vi "Get Control Reference.vi"(8 "error in":errorcluster, 9 "Control Label":string, 11 "Front Panel Reference In":refnum<vi>) -> (0 "error out":errorcluster, 1 "Selected Control Reference":refnum<vi>, 2 "Control References Array":refnum<vi>[](array[refnum]), 3 "Front Panel Reference Out":refnum<vi>)   [LabVIEW 2017, in "DTacq Plot Display Library.lvlib"]
uses:
  DTacq Plot Display Library.lvlib
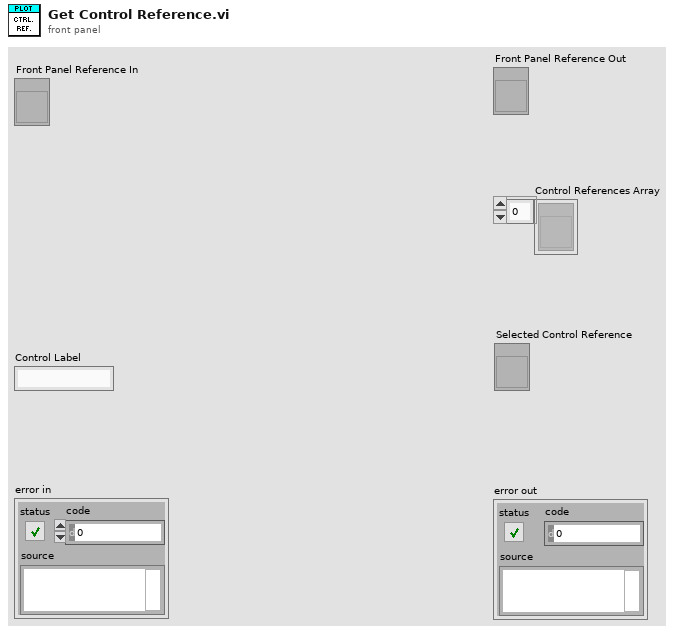
[diagram p1: front panel]
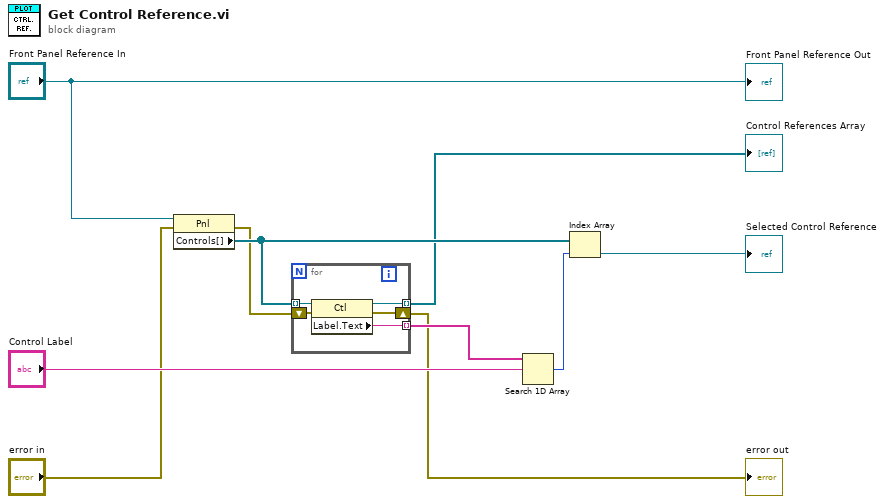
[diagram p0: block diagram]
diagram:
  n1 = property class="Pnl"(reference="Front Panel Reference In", error in="error in") -> (error out=w4:errorcluster, "Controls[]"=w9:refnum<vi>[])  [unwired: 1 out]
  n2 = for {
    tunnel: w9 -> [w15] mode=indexing
    tunnel: [w14] -> w7 mode=indexing
    shift-right: [w12] -> w2
    shift-left: w4 -> [w13]
    tunnel: [w11] -> w3 mode=indexing
    n3 = property class="Ctl"(reference=w15, error in=w13) -> (reference out=w11:refnum<vi>, error out=w12:errorcluster, "Label.Text"=w14:string)
  }
  "Control References Array" <- w3
  "error out" <- w2
  n4 = Search 1D Array(1D array=w7, element="Control Label") -> (index of element=w10:i32)  [unwired: 1 in]
  n5 = Index Array(array=w9, index=w10) -> (element=→"Selected Control Reference":refnum<vi>)
  "Front Panel Reference Out" <- "Front Panel Reference In"
